vi "SPI Write Read Bytes Of Event.vi"(0 "DevHandle":i32, 1 "pReadData":u8[](array[numeric])=array[4097 elements], 2 "IntervalTimeUs":i32, 3 "EventType":u8, 5 "SPIIndex":i32, 7 "pWriteData":u8[](array[numeric])=array[4097 elements], 9 "WriteLen":i32, 12 "ReadLen":i32, 13 "EventPin":i32, 14 "TimeOutOfMs":i32) -> (4 "pReadData out":u8[](array[numeric]), 6 "function return":i32, 8 "pWriteData out":u8[](array[numeric]))   [LabVIEW 2010, in "usb2spi.lvlib"]
doc: "int WINAPI SPI_WriteReadBytesOfEvent(int DevHandle,int SPIIndex,unsigned char *pWriteData,int WriteLen,unsigned char *pReadData,int ReadLen,int IntervalTimeUs,int EventPin,unsigned char EventType,int TimeOutOfMs);"
uses:
  usb2spi.lvlib
  USB2XXX/trunk/USB2XXX/USB2XXX/vs2019/Release/USB2XXX.dll
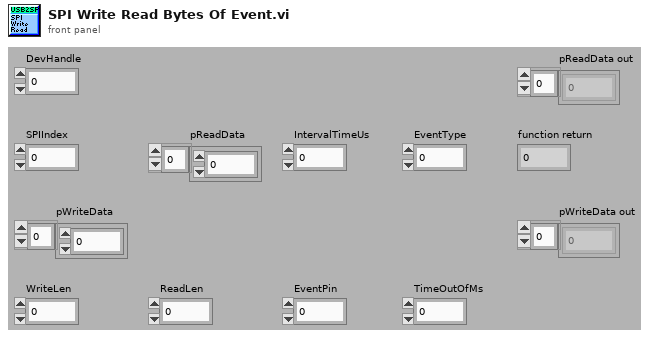
[diagram p1: front panel]
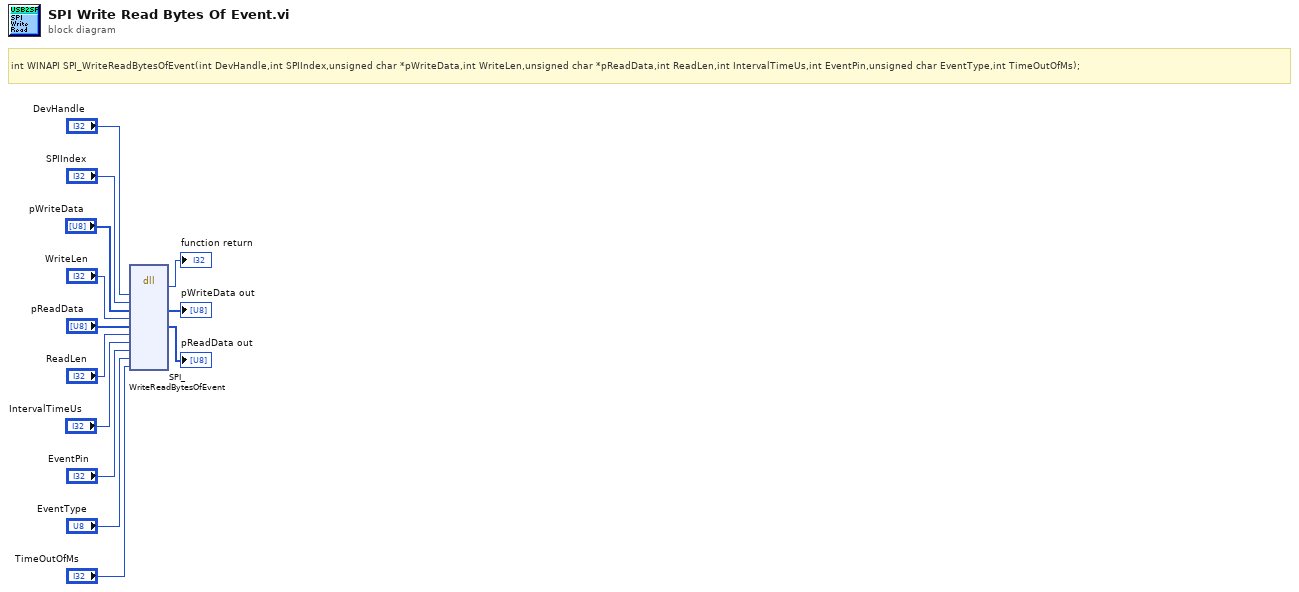
[diagram p0: block diagram]
diagram:
  # "int WINAPI SPI_WriteReadBytesOfEvent(int DevHandle,int SPIIndex,unsigned char *pWriteData,int WriteLen,unsigned char *pReadData,int ReadLen,int IntervalTimeUs,int EventPin,unsigned char EventType,int TimeOutOfMs);"
  n1 = dll-call lib="E:/Projects/USB2XXX/trunk/USB2XXX/USB2XXX/vs2019/Release/USB2XXX.*" fn="SPI_WriteReadBytesOfEvent"("DevHandle"="DevHandle", "SPIIndex"="SPIIndex", "pWriteData"="pWriteData", "WriteLen"="WriteLen", "pReadData"="pReadData", "ReadLen"="ReadLen", "IntervalTimeUs"="IntervalTimeUs", "EventPin"="EventPin", "EventType"="EventType", "TimeOutOfMs"="TimeOutOfMs") -> (→"function return":i32, "pWriteData"=→"pWriteData out":u8[], "pReadData"=→"pReadData out":u8[])  [unwired: 11 in, 2 out]
